vi "ChangeGate.vi"(1 "Current State":bool=TRUE, 2 "Previous State":bool=TRUE) -> (0 "Make a change":bool=TRUE)   [LabVIEW 2016]
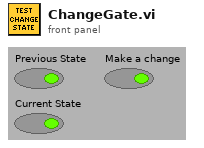
[diagram p1: front panel]
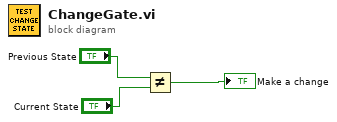
[diagram p0: block diagram]
diagram:
  n1 = Not Equal?(x="Previous State", y="Current State") -> (x != y?=→"Make a change":bool)
